vi "vi.CallLabVIEWType.vi"(8 "error in (no error)":errorcluster, 10 "LabVIEW Call":T1, 11 "User Data":variant) -> (0 "error out":errorcluster, 3 "Return Data":variant)   [LabVIEW 2014, in "GLue.lvlib" / "class.GLue.lvclass"]
uses:
  class.GLue.lvclass
  typedef.LVCallData.ctl
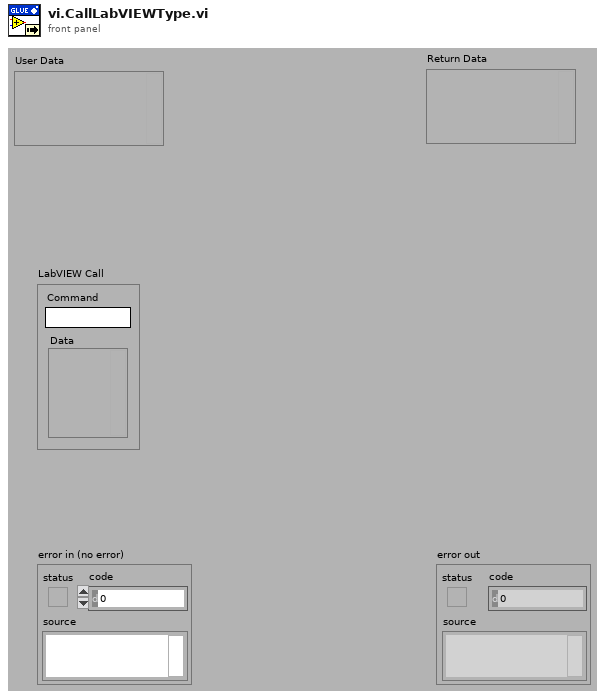
[diagram p1: front panel]
types:
  T1 = typedef "GLue.lvlib/class.GLue.lvclass/typedef.LVCallData.ctl" = cluster{"Command":string, "Data":variant}
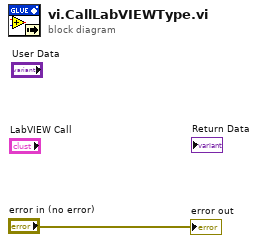
[diagram p0: block diagram]
diagram:
  "error out" <- "error in (no error)"
